vi "json tokenize.vi"(11 "String":string) -> (2 "error":bool, 3 "tokens":T1[](array[typedef]))   [LabVIEW 2014]
uses:
  json token.ctl
  json node type.ctl
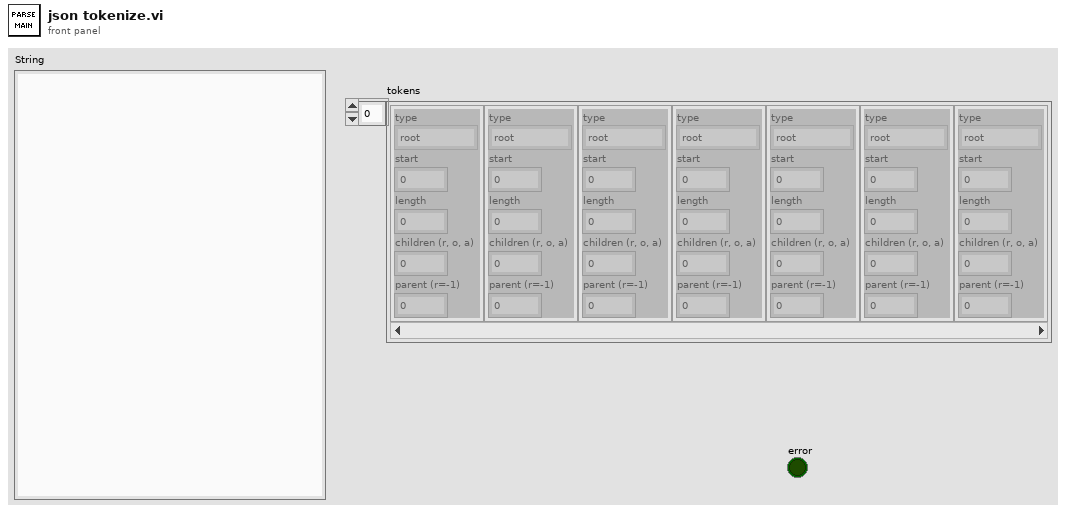
[diagram p1: front panel]
types:
  T1 = typedef "json token.ctl" = cluster{"type":T2, "start":i32, "length":i32, "children (r, o, a)":u16, "parent (r=-1)":i32}
  T2 = typedef "json node type.ctl" = enum16{"root", "object", "array", "number", "string value", "string key", "true", "false", "null"}
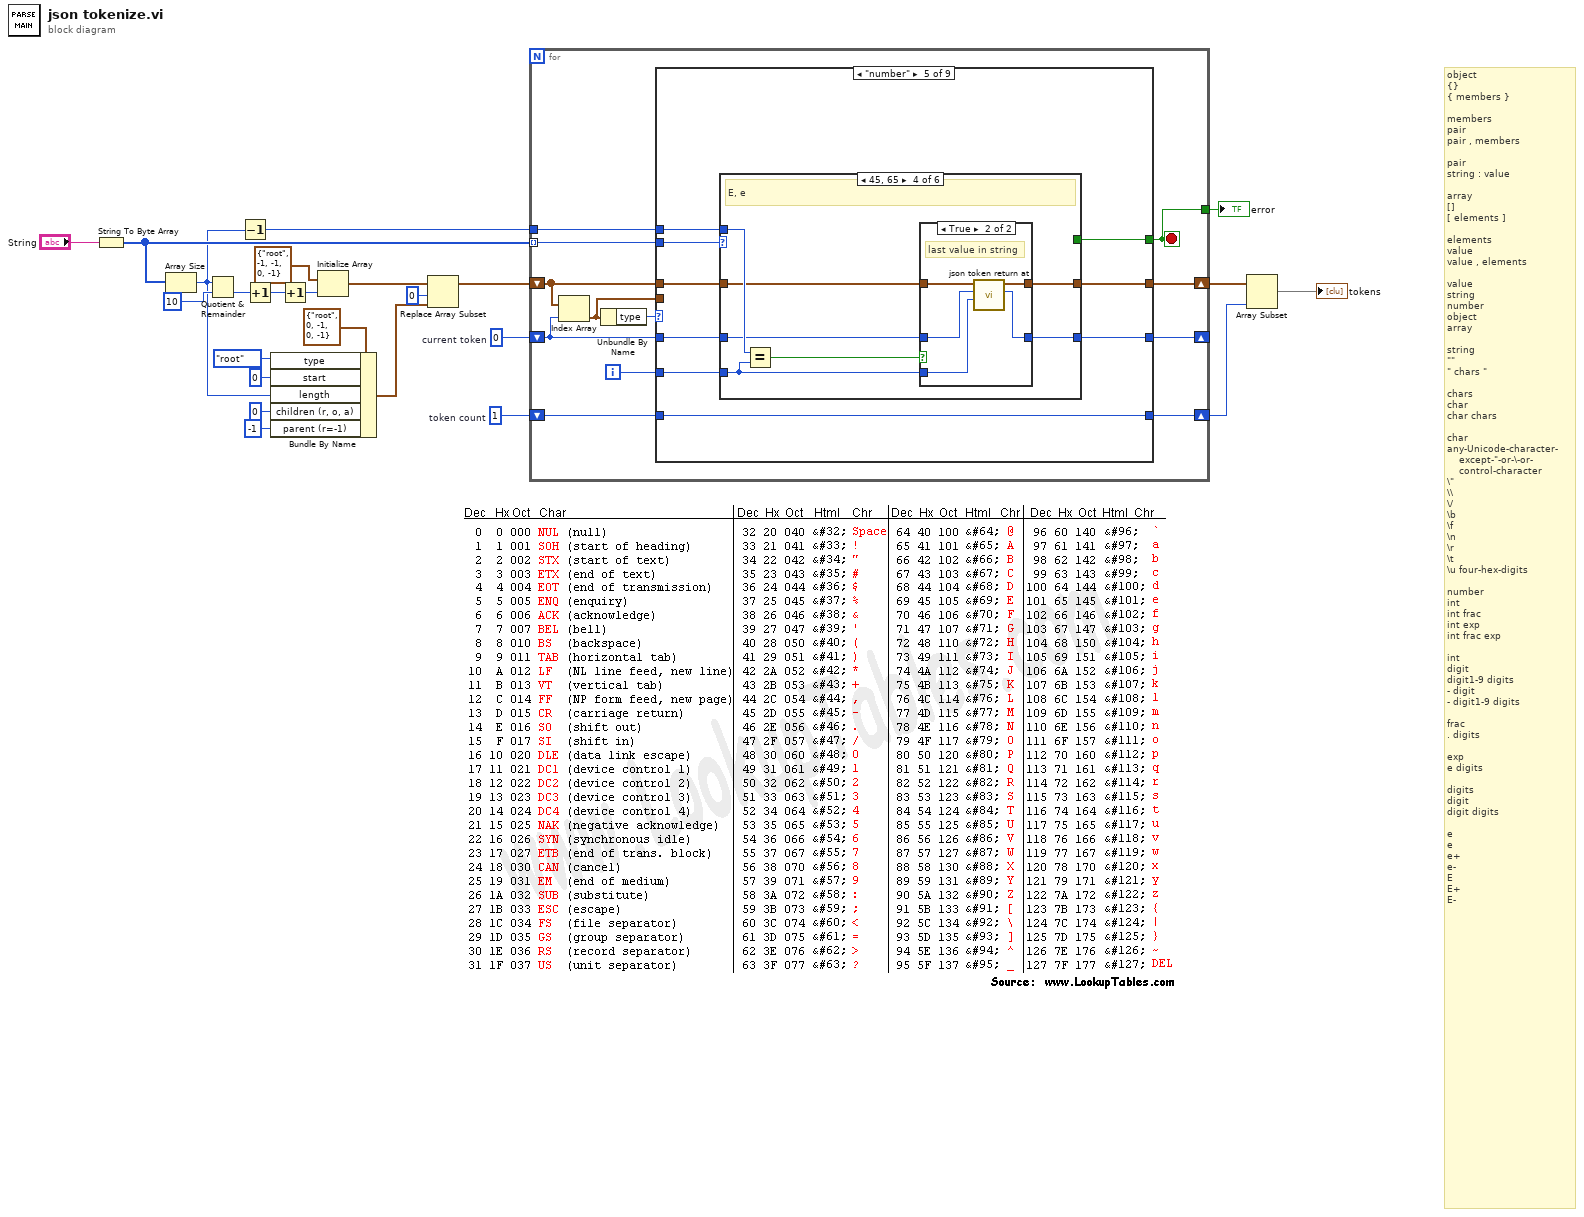
[diagram p0: block diagram]
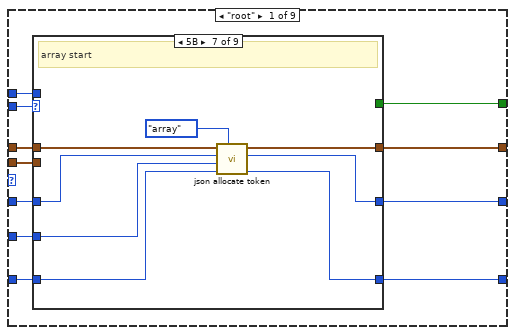
[diagram p2: hidden frame]
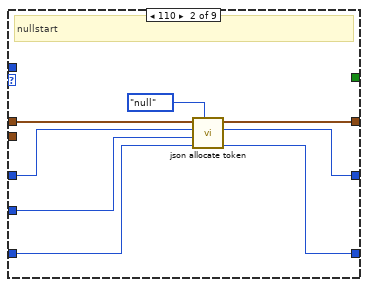
[diagram p4: hidden frame]
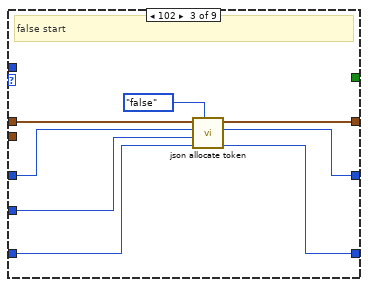
[diagram p5: hidden frame]
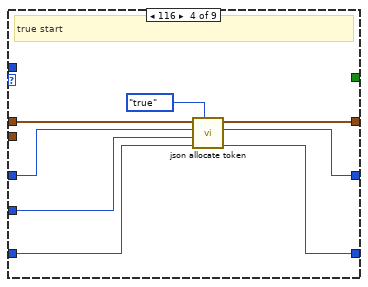
[diagram p6: hidden frame]
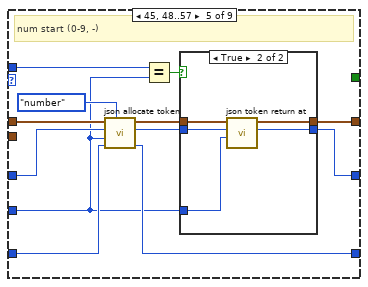
[diagram p7: hidden frame]
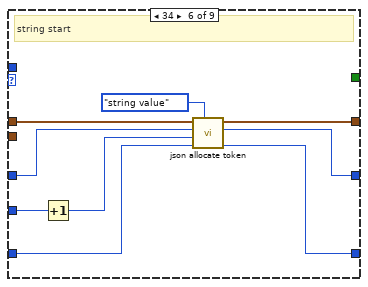
[diagram p9: hidden frame]
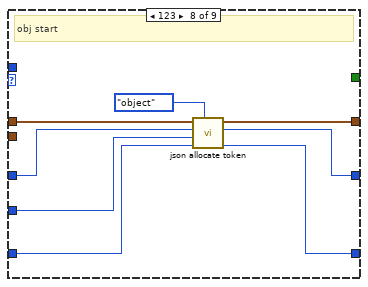
[diagram p10: hidden frame]
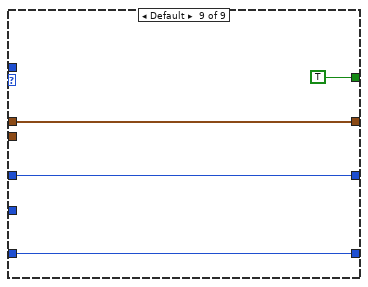
[diagram p11: hidden frame]
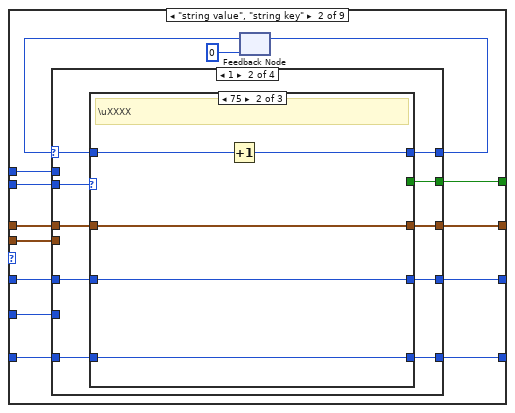
[diagram p12: hidden frame]
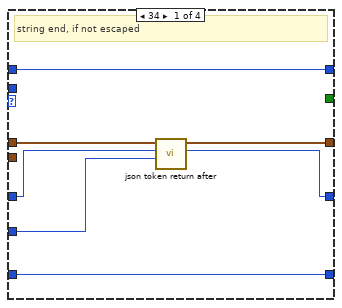
[diagram p14: hidden frame]
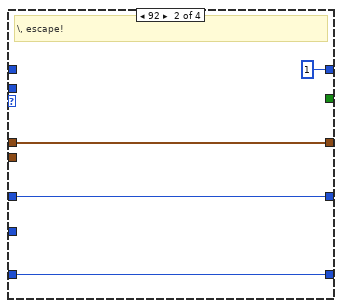
[diagram p15: hidden frame]
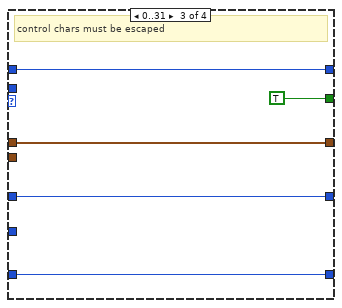
[diagram p16: hidden frame]
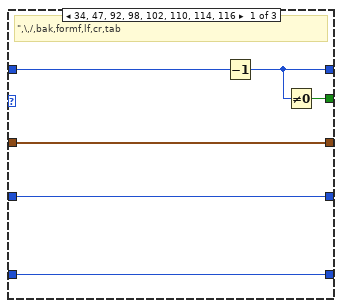
[diagram p17: hidden frame]
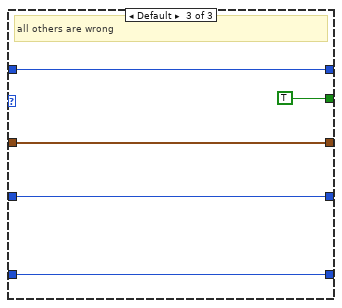
[diagram p18: hidden frame]
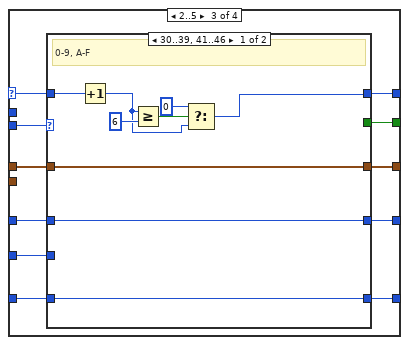
[diagram p19: hidden frame]
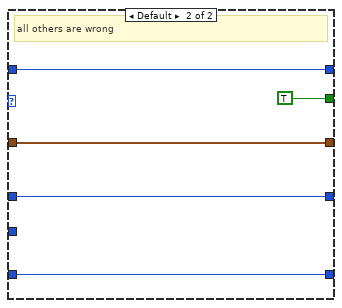
[diagram p20: hidden frame]
diagram:
  w9 = 1  # token count
  w19 = 0  # current token
  # "object\n{}\n{ members }\n\nmembers\npair\npair , members\n\npair\nstring : value\n\narray\n[]\n[ elements ]\n\nelements\nvalue \nvalue , elements\n\nvalue\nstring\nnumber\nobject\narray\n\nstring\n\"\"\n\" chars \"\n\nchars\nchar\nchar chars\n\nchar\nany-Unicode-character-\n    except-\"-or-\\-or-\n    control-character\n\\\"\n\\\\\n\\/\n\\b\n\\f\n\\n\n\\r\n\\t\n\\u four-hex-digits\n\nnumber\nint\nint frac\nint exp\nint frac exp\n\nint\ndigit\ndigit1-9 digits \n- digit\n- digit1-9 digits\n\nfrac\n. digits\n\nexp\ne digits\n\ndigits\ndigit\ndigit digits\n\ne\ne\ne+\ne-\nE\nE+\nE-"
  n1 = String To Byte Array(string="String") -> (unsigned byte array=w18:u8[])
  n2 = Array Size(array=w18) -> (size(s)=w4:i32)
  n3 = Quotient & Remainder(x=w4, y=10) -> (floor(x/y)=w22:i32)  [unwired: 1 out]
  n4 = Decrement(x=w4) -> (x-1=w3:i32)
  n5 = Increment(x=w22) -> (x+1=w8:i32)
  n6 = Bundle By Name(cluster=T1 {"type"=enum."root", "start"=0, "length"=-1, "children (r, o, a)"=0, "parent (r=-1)"=-1} ("token 2"), "type"=json_node_type."root", "start"=0, "length"=w4, "children (r, o, a)"=u16 0, "parent (r=-1)"=-1) -> (w10:T1)
  n7 = Increment(x=w8) -> (x+1=w1:i32)
  n8 = Initialize Array(T1 {"type"=enum."root", "start"=-1, "length"=-1, "children (r, o, a)"=0, "parent (r=-1)"=-1} ("token 2"), w1) -> (w20:T1[])
  n9 = Replace Array Subset(array=w20, new element=w10, index=0) -> (w17:T1[])
  n10 = for {
    shift-right: [w29] -> w7
    shift-left: w17 -> [w34]
    shift-right: [w27] -> _
    shift-left: w19 -> [w33]
    tunnel: w18 -> [w35] mode=indexing
    shift-right: [w31] -> w6
    shift-left: w9 -> [w32]
    tunnel: w3 -> [w26]
    tunnel: [w25] -> w2
    i -> [w28]
    stop <- w25 stop-if-true
    n11 = Index Array(array=w34, index=w33) -> (element=w30:T1)
    n12 = Unbundle By Name(w30) -> ("type"=w36:T2)
    n13 = case shown="\"number\"" w36 {
      tunnel: w35 -> [w47 w136 w227 w371 w452 w518 w553 w593 _]
      tunnel: [w43 w132 w234 w367 w451 w522 w557 w597 w626] -> w29
      tunnel: w34 -> [w44 w133 w235 w368 w450 w521 w556 w596 w626]
      tunnel: w33 -> [w45 w134 w231 w369 w449 w519 w554 w594 w625]
      tunnel: [w46 w135 w232 w370 w448 w520 w555 w595 w625] -> w27
      tunnel: w32 -> [w42 w131 w230 w366 w453 w525 w560 w600 w624]
      tunnel: w28 -> [w41 w130 w228 w365 w447 w514 w549 w589 _]
      tunnel: [w40 w129 w229 w364 w453 w525 w560 w600 w624] -> w31
      tunnel: [w39 w128 w233 w363 w445 w517 w552 w592 _] -> w25
      tunnel: w30 -> [w38 w127 w238 w362 _ w524 w559 w599 _]
      tunnel: w26 -> [w37 w126 _ _ w446 _ _ _ _]
      frame "root" {
        n14 = case shown="5B" w47 {
          tunnel: [w50 w53 w61 w69 w77 w97 w105 w113 w121] -> w46
          tunnel: w45 -> [w50 w56 w64 w72 w85 w100 w108 w116 w121]
          tunnel: w44 -> [w49 w58 w66 w74 w86 w102 w110 w118 w122]
          tunnel: [w49 w57 w65 w73 w78 w101 w109 w117 w122] -> w43
          tunnel: w42 -> [w48 w54 w62 w70 w84 w98 w106 w114 w120]
          tunnel: w41 -> [_ w55 w63 w71 w75 w99 w107 w115 _]
          tunnel: [w48 w52 w60 w68 w79 w96 w104 w112 w120] -> w40
          tunnel: [_ _ _ _ _ _ _ _ TRUE] -> w39
          tunnel: w38 -> [_ _ _ _ _ _ _ _ _]
          tunnel: w37 -> [_ _ _ _ w82 _ _ _ _]
          frame 9, 10, 13, 32 {
            # "whitespace"
          }
          frame 110 {
            # "nullstart"
            n15 = call "json allocate token.vi"("type"=json_node_type."null", "token count in"=w54, "start"=w55, "parent token"=w56, "tokens in"=w58) -> ("token count out"=w52:i32, "current token out"=w53:i32, "tokens out"=w57:T1[])  [unwired: 4 in]
          }
          frame 102 {
            # "false start"
            n16 = call "json allocate token.vi"("type"=json_node_type."false", "token count in"=w62, "start"=w63, "parent token"=w64, "tokens in"=w66) -> ("token count out"=w60:i32, "current token out"=w61:i32, "tokens out"=w65:T1[])  [unwired: 4 in]
          }
          frame 116 {
            # "true start"
            n17 = call "json allocate token.vi"("type"=json_node_type."true", "token count in"=w70, "start"=w71, "parent token"=w72, "tokens in"=w74) -> ("token count out"=w68:i32, "current token out"=w69:i32, "tokens out"=w73:T1[])  [unwired: 4 in]
          }
          frame 45, 48..57 {
            # "num start (0-9, -)"
            n18 = call "json allocate token.vi"("type"=json_node_type."number", "token count in"=w84, "start"=w75, "parent token"=w85, "tokens in"=w86) -> ("token count out"=w79:i32, "current token out"=w76:i32, "tokens out"=w80:T1[])  [unwired: 4 in]
            n19 = Equal?(x=w82, y=w75) -> (x = y?=w81:bool)
            n20 = case shown="True" w81 {
              tunnel: w80 -> [w88 w93]
              tunnel: [w88 w92] -> w78
              tunnel: [w87 w91] -> w77
              tunnel: w76 -> [w87 w90]
              tunnel: w75 -> [_ w89]
              frame False {
              }
              frame True {
                n21 = call "json token return at.vi"("string index"=w89, "token in"=w90, "tokens in"=w93) -> ("token out"=w91:i32, "tokens out"=w92:T1[])  [unwired: 7 in]
              }
            }
          }
          frame 34 {
            # "string start"
            n22 = Increment(x=w99) -> (x+1=w94:i32)
            n23 = call "json allocate token.vi"("type"=json_node_type."string value", "token count in"=w98, "start"=w94, "parent token"=w100, "tokens in"=w102) -> ("token count out"=w96:i32, "current token out"=w97:i32, "tokens out"=w101:T1[])  [unwired: 4 in]
          }
          frame 91 {
            # "array start"
            n24 = call "json allocate token.vi"("type"=json_node_type."array", "token count in"=w106, "start"=w107, "parent token"=w108, "tokens in"=w110) -> ("token count out"=w104:i32, "current token out"=w105:i32, "tokens out"=w109:T1[])  [unwired: 4 in]
          }
          frame 123 {
            # "obj start"
            n25 = call "json allocate token.vi"("type"=json_node_type."object", "token count in"=w114, "start"=w115, "parent token"=w116, "tokens in"=w118) -> ("token count out"=w112:i32, "current token out"=w113:i32, "tokens out"=w117:T1[])  [unwired: 4 in]
          }
          frame Default {
          }
        }
      }
      frame "string value", "string key" {
        n26 = feedback #1(u8 0) -> (w124:u8)
        n27 = case shown="1" w124 {
          selector: w124 -> [w138 w172 w198 w222]
          tunnel: w136 -> [w149 w173 w199 _]
          tunnel: [w148 w176 w202 w225] -> w135
          tunnel: w134 -> [w147 w177 w203 w225]
          tunnel: w133 -> [w146 w174 w200 w224]
          tunnel: [w145 w175 w201 w224] -> w132
          tunnel: w131 -> [w144 w178 w205 w223]
          tunnel: w130 -> [w143 _ w204 _]
          tunnel: [w142 w179 w206 w223] -> w129
          tunnel: [w141 w170 w196 TRUE] -> w128
          tunnel: w127 -> [w140 _ _ _]
          tunnel: w126 -> [w139 _ _ _]
          tunnel: [w137 w171 w197 w222] -> w125
          frame 0 {
            n28 = case shown="Default" w149 {
              tunnel: [w154 w160 w164 w169] -> w148
              tunnel: w147 -> [w152 w160 w164 w169]
              tunnel: w146 -> [w156 w159 w165 w168]
              tunnel: [w155 w159 w165 w168] -> w145
              tunnel: w144 -> [w151 w158 w163 w167]
              tunnel: w143 -> [w153 _ _ _]
              tunnel: [w151 w158 w163 w167] -> w142
              tunnel: [_ _ TRUE _] -> w141
              tunnel: w140 -> [_ _ _ _]
              tunnel: w139 -> [_ _ _ _]
              tunnel: w138 -> [w150 _ w161 w166]
              tunnel: [w150 u8 1 w161 w166] -> w137
              frame 34 {
                # "string end, if not escaped"
                n29 = call "json token return after.vi"("string index"=w153, "token in"=w152, "tokens in"=w156) -> ("token out"=w154:i32, "tokens out"=w155:T1[])  [unwired: 7 in]
              }
              frame 92 {
                # "\\, escape!"
              }
              frame 0..31 {
                # "control chars must be escaped"
              }
              frame Default {
                # "all others are OK"
              }
            }
          }
          frame 1 {
            n30 = case shown="75" w173 {
              tunnel: [w180 w186 w195] -> w176
              tunnel: w177 -> [w180 w186 w195]
              tunnel: w174 -> [w181 w187 w194]
              tunnel: [w181 w187 w194] -> w175
              tunnel: w178 -> [w185 w190 w193]
              tunnel: [w185 w190 w193] -> w179
              tunnel: [w183 _ TRUE] -> w170
              tunnel: w172 -> [w184 w189 w192]
              tunnel: [w182 w188 w192] -> w171
              frame 34, 47, 92, 98, 102, 110, 114, 116 {
                # "\",\\,/,bak,formf,lf,cr,tab"
                n31 = Decrement(x=w184) -> (x-1=w182:u8)
                n32 = Not Equal To 0?(x=w182) -> (x != 0?=w183:bool)
              }
              frame 117 {
                # "\\uXXXX"
                n33 = Increment(x=w189) -> (x+1=w188:u8)
              }
              frame Default {
                # "all others are wrong"
              }
            }
          }
          frame 2..5 {
            n34 = case shown="30..39, 41..46" w199 {
              tunnel: [w215 w220] -> w202
              tunnel: w203 -> [w215 w220]
              tunnel: w200 -> [w214 w219]
              tunnel: [w214 w219] -> w201
              tunnel: w205 -> [w213 w218]
              tunnel: w204 -> [_ _]
              tunnel: [w213 w218] -> w206
              tunnel: [_ TRUE] -> w196
              tunnel: w198 -> [w212 w217]
              tunnel: [w207 w217] -> w197
              frame 48..57, 65..70 {
                # "0-9, A-F"
                n35 = Increment(x=w212) -> (x+1=w209:u8)
                n36 = Greater Or Equal?(x=w209, y=u8 6) -> (x >= y?=w210:bool)
                n37 = Select(t=u8 0, s=w210, f=w209) -> (s? t:f=w207:u8)
              }
              frame Default {
                # "all others are wrong"
              }
            }
          }
          frame 6.. {
          }
        }
        n38 = feedback-in #1(w125) -> ()
      }
      frame "object" {
        n39 = Unbundle By Name(w238) -> ("children (r, o, a)"=w226:u16)
        n40 = And(x=w226, y=u16 1) -> (x .and. y?=w236:u16)
        n41 = case shown="0" w236 {
          tunnel: w235 -> [w242 w251 w284]
          tunnel: [w242 w249 w288] -> w234
          tunnel: [TRUE w250 w287] -> w233
          tunnel: [w240 w248 w286] -> w232
          tunnel: w231 -> [w240 w244 w283]
          tunnel: w230 -> [w239 w246 w281]
          tunnel: [w239 w247 w285] -> w229
          tunnel: w228 -> [_ w245 w282]
          tunnel: w227 -> [_ w252 w280]
          tunnel: w226 -> [_ w243 _]
          frame Default {
            # "magic"
          }
          frame 0 {
            # "even, looking for next key"
            n42 = case shown="7D" w252 {
              tunnel: [w255 w260 w265 w272 w278] -> w248
              tunnel: w244 -> [w255 w260 w267 w271 w278]
              tunnel: w251 -> [w254 w259 w269 w274 w279]
              tunnel: [w254 w259 w268 w273 w279] -> w249
              tunnel: w246 -> [w253 w258 w266 w275 w277]
              tunnel: w245 -> [_ _ w262 w270 _]
              tunnel: [w253 w258 w264 w275 w277] -> w247
              tunnel: [_ w256 _ _ TRUE] -> w250
              tunnel: w243 -> [_ w257 _ _ _]
              frame 9, 10, 13, 32 {
                # "whitespace"
              }
              frame 44 {
                # "comma"
                n43 = Equal To 0?(x=w257) -> (x = 0?=w256:bool)
              }
              frame 34 {
                # "string key start"
                n44 = Increment(x=w262) -> (x+1=w261:i32)
                n45 = call "json allocate token.vi"("type"=json_node_type."string key", "token count in"=w266, "start"=w261, "parent token"=w267, "tokens in"=w269) -> ("token count out"=w264:i32, "current token out"=w265:i32, "tokens out"=w268:T1[])  [unwired: 4 in]
              }
              frame 125 {
                n46 = call "json token return at.vi"("string index"=w270, "token in"=w271, "tokens in"=w274) -> ("token out"=w272:i32, "tokens out"=w273:T1[])  [unwired: 7 in]
              }
              frame Default {
              }
            }
          }
          frame 1 {
            # "odd, looking for next value"
            n47 = case shown="7D" w280 {
              tunnel: [w291 w294 w297 w305 w313 w321 w330 w338 w346 w355 w360] -> w286
              tunnel: w283 -> [w291 w294 w300 w308 w316 w324 w333 w341 w349 w354 w360]
              tunnel: w284 -> [w290 w293 w302 w310 w318 w326 w335 w343 w351 w357 w361]
              tunnel: [w290 w293 w301 w309 w317 w325 w334 w342 w350 w356 w361] -> w288
              tunnel: w281 -> [w289 w292 w298 w306 w314 w322 w331 w339 w347 w353 w359]
              tunnel: w282 -> [_ _ w299 w307 w315 w323 w332 w340 w348 w352 _]
              tunnel: [w289 w292 w296 w304 w312 w320 w329 w337 w345 w353 w359] -> w285
              tunnel: [_ _ _ _ _ _ _ _ _ _ TRUE] -> w287
              frame 9, 10, 13, 32 {
                # "whitespace"
              }
              frame 58 {
                # "colon"
              }
              frame 110 {
                # "nullstart"
                n48 = call "json allocate token.vi"("type"=json_node_type."null", "token count in"=w298, "start"=w299, "parent token"=w300, "tokens in"=w302) -> ("token count out"=w296:i32, "current token out"=w297:i32, "tokens out"=w301:T1[])  [unwired: 4 in]
              }
              frame 102 {
                # "false start"
                n49 = call "json allocate token.vi"("type"=json_node_type."false", "token count in"=w306, "start"=w307, "parent token"=w308, "tokens in"=w310) -> ("token count out"=w304:i32, "current token out"=w305:i32, "tokens out"=w309:T1[])  [unwired: 4 in]
              }
              frame 116 {
                # "true start"
                n50 = call "json allocate token.vi"("type"=json_node_type."true", "token count in"=w314, "start"=w315, "parent token"=w316, "tokens in"=w318) -> ("token count out"=w312:i32, "current token out"=w313:i32, "tokens out"=w317:T1[])  [unwired: 4 in]
              }
              frame 45, 48..57 {
                # "num start (0-9, -)"
                n51 = call "json allocate token.vi"("type"=json_node_type."number", "token count in"=w322, "start"=w323, "parent token"=w324, "tokens in"=w326) -> ("token count out"=w320:i32, "current token out"=w321:i32, "tokens out"=w325:T1[])  [unwired: 4 in]
              }
              frame 34 {
                # "string start"
                n52 = Increment(x=w332) -> (x+1=w327:i32)
                n53 = call "json allocate token.vi"("type"=json_node_type."string value", "token count in"=w331, "start"=w327, "parent token"=w333, "tokens in"=w335) -> ("token count out"=w329:i32, "current token out"=w330:i32, "tokens out"=w334:T1[])  [unwired: 4 in]
              }
              frame 91 {
                # "array start"
                n54 = call "json allocate token.vi"("type"=json_node_type."array", "token count in"=w339, "start"=w340, "parent token"=w341, "tokens in"=w343) -> ("token count out"=w337:i32, "current token out"=w338:i32, "tokens out"=w342:T1[])  [unwired: 4 in]
              }
              frame 123 {
                # "obj start"
                n55 = call "json allocate token.vi"("type"=json_node_type."object", "token count in"=w347, "start"=w348, "parent token"=w349, "tokens in"=w351) -> ("token count out"=w345:i32, "current token out"=w346:i32, "tokens out"=w350:T1[])  [unwired: 4 in]
              }
              frame 125 {
                # "obj end"
                n56 = call "json token return at.vi"("string index"=w352, "token in"=w354, "tokens in"=w357) -> ("token out"=w355:i32, "tokens out"=w356:T1[])  [unwired: 7 in]
              }
              frame Default {
              }
            }
          }
        }
      }
      frame "array" {
        n57 = case shown="22" w371 {
          tunnel: [w374 w377 w380 w388 w396 w404 w413 w421 w429 w438 w443] -> w370
          tunnel: w369 -> [w374 w377 w383 w391 w399 w407 w416 w424 w432 w437 w443]
          tunnel: w368 -> [w373 w376 w385 w393 w401 w409 w418 w426 w434 w440 w444]
          tunnel: [w373 w376 w384 w392 w400 w408 w417 w425 w433 w439 w444] -> w367
          tunnel: w366 -> [w372 w375 w381 w389 w397 w405 w414 w422 w430 w436 w442]
          tunnel: w365 -> [_ _ w382 w390 w398 w406 w415 w423 w431 w435 _]
          tunnel: [w372 w375 w379 w387 w395 w403 w412 w420 w428 w436 w442] -> w364
          tunnel: [_ _ _ _ _ _ _ _ _ _ TRUE] -> w363
          tunnel: w362 -> [_ _ _ _ _ _ _ _ _ _ _]
          frame 9, 10, 13, 32 {
            # "whitespace"
          }
          frame 44 {
            # "comma"
          }
          frame 110 {
            # "nullstart"
            n58 = call "json allocate token.vi"("type"=json_node_type."null", "token count in"=w381, "start"=w382, "parent token"=w383, "tokens in"=w385) -> ("token count out"=w379:i32, "current token out"=w380:i32, "tokens out"=w384:T1[])  [unwired: 4 in]
          }
          frame 102 {
            # "false start"
            n59 = call "json allocate token.vi"("type"=json_node_type."false", "token count in"=w389, "start"=w390, "parent token"=w391, "tokens in"=w393) -> ("token count out"=w387:i32, "current token out"=w388:i32, "tokens out"=w392:T1[])  [unwired: 4 in]
          }
          frame 116 {
            # "true start"
            n60 = call "json allocate token.vi"("type"=json_node_type."true", "token count in"=w397, "start"=w398, "parent token"=w399, "tokens in"=w401) -> ("token count out"=w395:i32, "current token out"=w396:i32, "tokens out"=w400:T1[])  [unwired: 4 in]
          }
          frame 45, 48..57 {
            # "num start (0-9, -)"
            n61 = call "json allocate token.vi"("type"=json_node_type."number", "token count in"=w405, "start"=w406, "parent token"=w407, "tokens in"=w409) -> ("token count out"=w403:i32, "current token out"=w404:i32, "tokens out"=w408:T1[])  [unwired: 4 in]
          }
          frame 34 {
            # "string start"
            n62 = Increment(x=w415) -> (x+1=w410:i32)
            n63 = call "json allocate token.vi"("type"=json_node_type."string value", "token count in"=w414, "start"=w410, "parent token"=w416, "tokens in"=w418) -> ("token count out"=w412:i32, "current token out"=w413:i32, "tokens out"=w417:T1[])  [unwired: 4 in]
          }
          frame 91 {
            # "array start"
            n64 = call "json allocate token.vi"("type"=json_node_type."array", "token count in"=w422, "start"=w423, "parent token"=w424, "tokens in"=w426) -> ("token count out"=w420:i32, "current token out"=w421:i32, "tokens out"=w425:T1[])  [unwired: 4 in]
          }
          frame 123 {
            # "obj start"
            n65 = call "json allocate token.vi"("type"=json_node_type."object", "token count in"=w430, "start"=w431, "parent token"=w432, "tokens in"=w434) -> ("token count out"=w428:i32, "current token out"=w429:i32, "tokens out"=w433:T1[])  [unwired: 4 in]
          }
          frame 93 {
            # "array end"
            n66 = call "json token return at.vi"("string index"=w435, "token in"=w437, "tokens in"=w440) -> ("token out"=w438:i32, "tokens out"=w439:T1[])  [unwired: 7 in]
          }
          frame Default {
          }
        }
      }
      frame "number" {
        n67 = case shown="45, 65" w452 {
          tunnel: [w457 w463 w478 w492 w505 w510] -> w451
          tunnel: w450 -> [w458 w464 w475 w489 w506 w513]
          tunnel: w449 -> [w455 w461 w474 w488 w504 w512]
          tunnel: [w456 w462 w477 w491 w503 w509] -> w448
          tunnel: w447 -> [w454 w460 w476 w490 w502 w507]
          tunnel: w446 -> [_ w466 w480 w494 _ _]
          tunnel: [TRUE _ _ _ _ _] -> w445
          frame Default {
            n68 = call "json token return after.vi"("string index"=w454, "token in"=w455, "tokens in"=w458) -> ("token out"=w456:i32, "tokens out"=w457:T1[])  [unwired: 7 in]
          }
          frame 43, 45, 48..57 {
            # "0-9, -, +"
            n69 = Equal?(x=w466, y=w460) -> (x = y?=w465:bool)
            n70 = case shown="True" w465 {
              tunnel: w464 -> [w468 w473]
              tunnel: [w468 w472] -> w463
              tunnel: [w467 w471] -> w462
              tunnel: w461 -> [w467 w470]
              tunnel: w460 -> [_ w469]
              frame False {
                # "keep going"
              }
              frame True {
                # "last value in string"
                n71 = call "json token return at.vi"("string index"=w469, "token in"=w470, "tokens in"=w473) -> ("token out"=w471:i32, "tokens out"=w472:T1[])  [unwired: 7 in]
              }
            }
          }
          frame 46 {
            # "."
            n72 = Equal?(x=w480, y=w476) -> (x = y?=w479:bool)
            n73 = case shown="True" w479 {
              tunnel: w475 -> [w482 w487]
              tunnel: [w482 w486] -> w478
              tunnel: [w481 w485] -> w477
              tunnel: w474 -> [w481 w484]
              tunnel: w476 -> [_ w483]
              frame False {
                # "keep going"
              }
              frame True {
                # "last value in string"
                n74 = call "json token return at.vi"("string index"=w483, "token in"=w484, "tokens in"=w487) -> ("token out"=w485:i32, "tokens out"=w486:T1[])  [unwired: 7 in]
              }
            }
          }
          frame 69, 101 {
            # "E, e"
            n75 = Equal?(x=w494, y=w490) -> (x = y?=w493:bool)
            n76 = case shown="True" w493 {
              tunnel: w489 -> [w496 w501]
              tunnel: [w496 w500] -> w492
              tunnel: [w495 w499] -> w491
              tunnel: w488 -> [w495 w498]
              tunnel: w490 -> [_ w497]
              frame False {
                # "keep going"
              }
              frame True {
                # "last value in string"
                n77 = call "json token return at.vi"("string index"=w497, "token in"=w498, "tokens in"=w501) -> ("token out"=w499:i32, "tokens out"=w500:T1[])  [unwired: 7 in]
              }
            }
          }
          frame 9, 10, 13, 32, 44 {
            # "whitespace, comma"
            n78 = call "json token return after.vi"("string index"=w502, "token in"=w504, "tokens in"=w506) -> ("token out"=w503:i32, "tokens out"=w505:T1[])  [unwired: 7 in]
          }
          frame 93, 125 {
            # "end obj or array"
            n79 = call "json token return after.vi"("string index"=w507, "token in"=w512, "tokens in"=w513) -> ("token out"=w508:i32, "tokens out"=w511:T1[])  [unwired: 7 in]
            n80 = call "json token return at.vi"("string index"=w507, "token in"=w508, "tokens in"=w511) -> ("token out"=w509:i32, "tokens out"=w510:T1[])  [unwired: 7 in]
          }
        }
      }
      frame "true" {
        n81 = Unbundle By Name(w524) -> ("parent (r=-1)"=w515:i32, "start"=w516:i32)
        n82 = Subtract(x=w514, y=w516) -> (x-y=w523:i32)
        n83 = case shown="3" w523 {
          tunnel: [w528 w530 w535 w540] -> w522
          tunnel: w521 -> [w528 w530 w535 w541]
          tunnel: [w527 w529 w534 w542] -> w520
          tunnel: w519 -> [w527 w529 w534 w539]
          tunnel: w518 -> [_ w533 w538 w545]
          tunnel: [FALSE w531 w536 w543] -> w517
          tunnel: w515 -> [_ _ _ w542]
          frame ..0, 4.. {
          }
          frame 1 {
            w532 = u8 114  # R
            n84 = Not Equal?(x=w533, y=w532) -> (x != y?=w531:bool)
          }
          frame 2 {
            w537 = u8 117  # U
            n85 = Not Equal?(x=w538, y=w537) -> (x != y?=w536:bool)
          }
          frame 3 {
            w544 = u8 101  # E
            n86 = in-place {
              n87 = in-place-array #2(w541, w539) -> (w548:T1)
              n88 = Bundle By Name(cluster=w548, "length"=4) -> (w547:T1)
              n89 = in-place-array #2(w547) -> (w540:T1[])  [unwired: 1 out]
            }
            n90 = Not Equal?(x=w545, y=w544) -> (x != y?=w543:bool)
          }
        }
      }
      frame "false" {
        n91 = Unbundle By Name(w559) -> ("parent (r=-1)"=w550:i32, "start"=w551:i32)
        n92 = Subtract(x=w549, y=w551) -> (x-y=w558:i32)
        n93 = case shown="4" w558 {
          tunnel: [w563 w565 w570 w575 w580] -> w557
          tunnel: w556 -> [w563 w565 w570 w575 w581]
          tunnel: [w562 w564 w569 w574 w582] -> w555
          tunnel: w554 -> [w562 w564 w569 w574 w579]
          tunnel: w553 -> [_ w568 w573 w578 w585]
          tunnel: [FALSE w566 w571 w576 w583] -> w552
          tunnel: w550 -> [_ _ _ _ w582]
          frame ..0, 5.. {
          }
          frame 1 {
            w567 = u8 97  # A
            n94 = Not Equal?(x=w568, y=w567) -> (x != y?=w566:bool)
          }
          frame 2 {
            w572 = u8 108  # L
            n95 = Not Equal?(x=w573, y=w572) -> (x != y?=w571:bool)
          }
          frame 3 {
            w577 = u8 115  # S
            n96 = Not Equal?(x=w578, y=w577) -> (x != y?=w576:bool)
          }
          frame 4 {
            w584 = u8 101  # E
            n97 = in-place {
              n98 = in-place-array #3(w581, w579) -> (w588:T1)
              n99 = Bundle By Name(cluster=w588, "length"=5) -> (w587:T1)
              n100 = in-place-array #3(w587) -> (w580:T1[])  [unwired: 1 out]
            }
            n101 = Not Equal?(x=w585, y=w584) -> (x != y?=w583:bool)
          }
        }
      }
      frame "null" {
        n102 = Unbundle By Name(w599) -> ("parent (r=-1)"=w590:i32, "start"=w591:i32)
        n103 = Subtract(x=w589, y=w591) -> (x-y=w598:i32)
        n104 = case shown="3" w598 {
          tunnel: [w603 w605 w610 w615] -> w597
          tunnel: w596 -> [w603 w605 w610 w616]
          tunnel: [w602 w604 w609 w617] -> w595
          tunnel: w594 -> [w602 w604 w609 w614]
          tunnel: w593 -> [_ w608 w613 w620]
          tunnel: [FALSE w606 w611 w618] -> w592
          tunnel: w590 -> [_ _ _ w617]
          frame ..0, 4.. {
          }
          frame 1 {
            w607 = u8 117  # U
            n105 = Not Equal?(x=w608, y=w607) -> (x != y?=w606:bool)
          }
          frame 2 {
            w612 = u8 108  # L
            n106 = Not Equal?(x=w613, y=w612) -> (x != y?=w611:bool)
          }
          frame 3 {
            w619 = u8 108  # L
            n107 = in-place {
              n108 = in-place-array #4(w616, w614) -> (w623:T1)
              n109 = Bundle By Name(cluster=w623, "length"=4) -> (w622:T1)
              n110 = in-place-array #4(w622) -> (w615:T1[])  [unwired: 1 out]
            }
            n111 = Not Equal?(x=w620, y=w619) -> (x != y?=w618:bool)
          }
        }
      }
      frame Default {
      }
    }
  }
  "error" <- w2
  n112 = Array Subset(array=w7, length=w6) -> (→"tokens":T1[])  [unwired: 1 in]
